vi "Run.vi"(8 "error in (no error)":errorcluster, 11 "HGF_Application in":refnum<class "HGF_Application.lvclass">) -> (0 "error out":errorcluster, 3 "HGF_Application out":refnum<class "HGF_Application.lvclass">)   [LabVIEW 2012, in "HGF_ApplicationBaseClasses.lvlib" / "HGF_Application.lvclass"]
uses:
  HGF_Application.lvclass
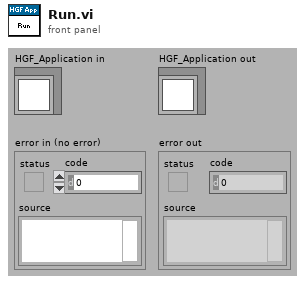
[diagram p1: front panel]
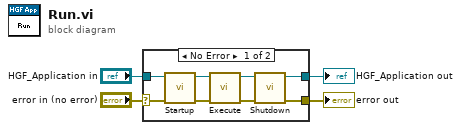
[diagram p0: block diagram]
diagram:
  n1 = case shown="No Error" "error in (no error)" {
    selector: "error in (no error)" -> [w6 w14]
    tunnel: [w5 w14] -> w3
    tunnel: [w9 w13] -> w1
    tunnel: "HGF_Application in" -> [w12 w13]
    frame No Error {
      n2 = call-dynamic "Startup.vi"("error in (no error)"=w6, "HGF_Application in"=w12) -> ("error out"=w7:errorcluster, "HGF_Application out"=w11:refnum<class "HGF_Application.lvclass">)  [unwired: 8 in]
      n3 = call-dynamic "Execute.vi"("error in (no error)"=w7, "HGF_Application in"=w11) -> ("error out"=w8:errorcluster, "HGF_Application out"=w10:refnum<class "HGF_Application.lvclass">)  [unwired: 8 in]
      n4 = call-dynamic "Shutdown.vi"("error in (no error)"=w8, "HGF_Application in"=w10) -> ("error out"=w5:errorcluster, "HGF_Application out"=w9:refnum<class "HGF_Application.lvclass">)  [unwired: 8 in]
    }
    frame Error {
    }
  }
  "error out" <- w3
  "HGF_Application out" <- w1
